vi "prac1-1.vi"(0 "Grados Farenheit":dbl) -> (1 "Grados Celcius":dbl(slide) scale=0.0..100.0, 2 "Grados Rankine":dbl(slide) scale=0.0..1000.0)   [LabVIEW 2014]
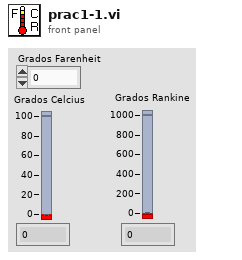
[diagram p1: front panel]
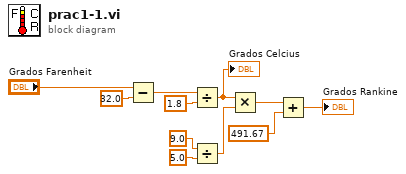
[diagram p0: block diagram]
diagram:
  n1 = Subtract(x="Grados Farenheit", y=32.0) -> (x-y=w10:dbl)
  n2 = Divide(x=w10, y=1.8) -> (x/y=w4:dbl)
  "Grados Celcius" <- w4
  n3 = Divide(x=9.0, y=5.0) -> (x/y=w5:dbl)
  n4 = Multiply(x=w4, y=w5) -> (x*y=w3:dbl)
  n5 = Add(x=w3, y=491.67) -> (x+y=→"Grados Rankine":dbl)
